vi "Build Result String.vi"(9 "Error":errorcluster, 10 "Abort?":bool, 11 "Pass?":bool) -> (3 "Result String":string)   [LabVIEW 2020, in "MacroAssert.lvlib"]
uses:
  MacroAssert.lvlib
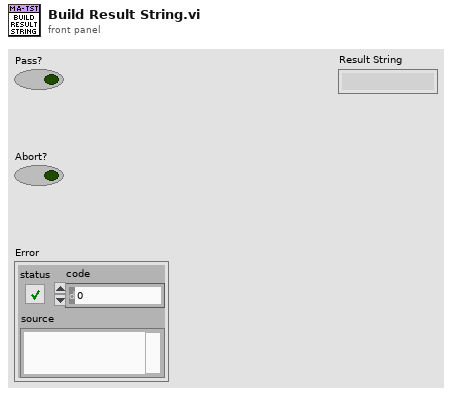
[diagram p1: front panel]
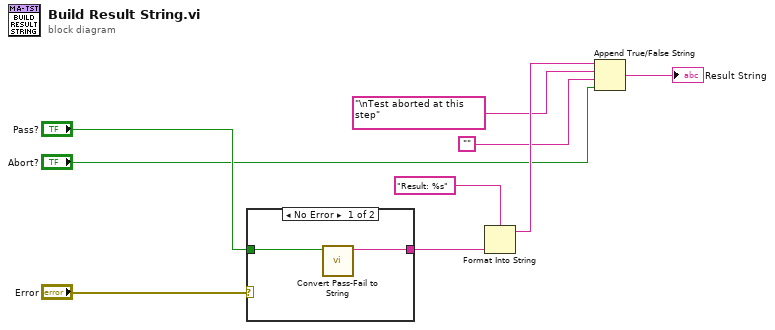
[diagram p0: block diagram]
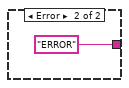
[diagram p2: hidden frame]
diagram:
  n1 = case shown="No Error" "Error" {
    tunnel: "Pass?" -> [w11 _]
    tunnel: [w10 "ERROR" ("Pass/Fail String")] -> w6
    frame No Error {
      n2 = call "Convert Pass-Fail to String.vi"("Pass?"=w11) -> ("Pass/Fail String"=w10:string)  [unwired: 10 in]
    }
    frame Error {
    }
  }
  n3 = Format Into String(format string="Result: %s", w6) -> (resulting string=w5:string)  [unwired: 2 in, 1 out]
  n4 = Append True/False String(1:"Abort?", 2:"", 3:"\nTest aborted at this step" ("true string"), 4:w5) -> (0:→"Result String":string)
